vi "Set Temp via Global Variables.vi"(1 "Rate":dbl=10.0, 2 "Temperature":dbl=300.0) -> ()   [LabVIEW 2013]
uses:
  PPMS Global.vi
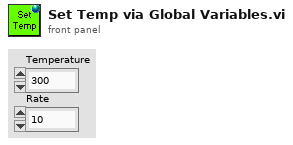
[diagram p1: front panel]
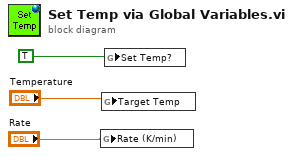
[diagram p0: block diagram]
diagram:
  n1 = global write "PPMS Global.vi" "Rate (K/min)"("Rate") -> ()
  n2 = global write "PPMS Global.vi" "Target Temp"("Temperature") -> ()
  n3 = global write "PPMS Global.vi" "Set Temp?"(TRUE ("Remote")) -> ()
